vi "set_CW_light_subvi.vi"(8 "error in (no error)":errorcluster, 9 "Num Bytes to Fetch (64) in":u8=64 min=1, 10 "Aardvark Handle":i32 min=0, 11 "Address (0x50) in":u16=80 max=1023 format="%.0x") -> (0 "error out":errorcluster)   [LabVIEW 2014]
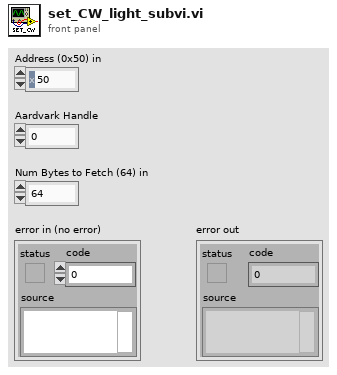
[diagram p1: front panel]
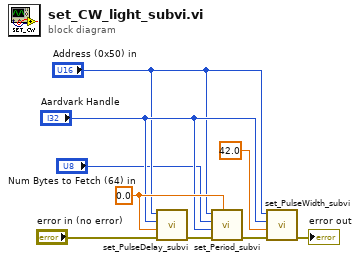
[diagram p0: block diagram]
diagram:
  w7 = 0.0
  n1 = call "set_PulseDelay_subvi.vi"("error in (no error)"="error in (no error)", "Pulse Delay"=w7, "Aardvark Handle"="Aardvark Handle", "Address (0x50) in"="Address (0x50) in") -> ("error out"=w8:errorcluster)  [unwired: 7 in]
  n2 = call "set_Period_subvi.vi"("Period"=w7, "error in (no error)"=w8, "Aardvark Handle"="Aardvark Handle", "Num Bytes to Fetch (64) in"="Num Bytes to Fetch (64) in", "Address (0x50) in"="Address (0x50) in") -> ("error out"=w6:errorcluster)  [unwired: 6 in]
  n3 = call "set_PulseWidth_subvi.vi"("error in (no error)"=w6, "Pulsewidth"=42.0, "Aardvark Handle"="Aardvark Handle", "Address (0x50) in"="Address (0x50) in") -> ("error out"=→"error out":errorcluster)  [unwired: 7 in]
